vi "ENA Validated Commands.vi"() -> ()   [LabVIEW 2013]
panel:
  out "Return Count":i32
  out "VISA resource name out":refnum<visa-resource-name>
  out "error out":errorcluster
  in  "error in (no error)":errorcluster
  in  "VISA resource name":refnum<visa-resource-name>
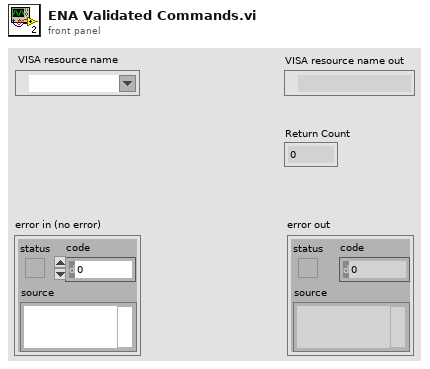
[diagram p1: front panel]
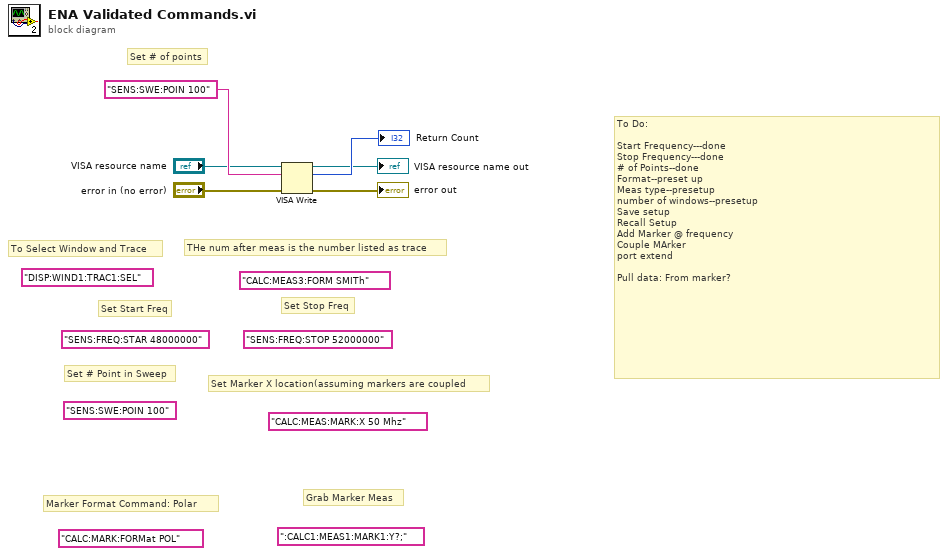
[diagram p0: block diagram]
diagram:
  (unwired) ":CALC1:MEAS1:MARK1:Y?;" ("write buffer")
  (unwired) "CALC:MARK:FORMat POL" ("write buffer")
  (unwired) "SENS:SWE:POIN 100" ("write buffer")
  (unwired) "CALC:MEAS:MARK:X 50 Mhz" ("write buffer")
  (unwired) "SENS:FREQ:STOP 52000000" ("write buffer")
  (unwired) "SENS:FREQ:STAR 48000000" ("write buffer")
  (unwired) "CALC:MEAS3:FORM SMITh" ("write buffer")
  (unwired) "DISP:WIND1:TRAC1:SEL" ("write buffer")
  # "Grab Marker Meas"
  # "Marker Format Command: Polar"
  # "Set # Point in Sweep"
  # "Set Marker X location(assuming markers are coupled"
  # "Set Stop Freq"
  # "Set Start Freq"
  # "THe num after meas is the number listed as trace"
  # "To Select Window and Trace"
  # "Set # of points"
  # "To Do:\n\nStart Frequency---done\nStop Frequency---done\n# of Points--done\nFormat--preset up\nMeas type--presetup\nnumber of windows--presetup\nSave setup\nRecall Setup\nAdd Marker @ frequency\nCouple MArker\nport extend\n\nPull data: From marker?"
  n1 = VISA Write(VISA resource name="VISA resource name", write buffer="SENS:SWE:POIN 100", error in (no error)="error in (no error)") -> (VISA resource name out=→"VISA resource name out":refnum<visa-resource-name>, return count=→"Return Count":u32, error out=→"error out":errorcluster)
